vi "Initialize Text Log File.vi"(8 "error in (no error)":errorcluster, 9 "Operation":T1, 10 "File Path":path, 11 "Text Log File Specification in":refnum<class "Text Log File Specification.lvclass">) -> (0 "error out":errorcluster, 1 "Log File out":refnum<class "Log File.lvclass">, 3 "Text Log File Specification out":refnum<class "Text Log File Specification.lvclass">)   [LabVIEW 2015, in "Text Log File Specification.lvclass"]
uses:
  Text Log File Specification.lvclass
  Logs/Log Files/Log File/Log File.lvclass
  Logs/Log Files/Log File/Operation.ctl
  Text Log File Specification.lvclass/Text Log File Specification.ctl
  Logs/Log Files/Text Log File/Text Log File.lvclass
  Logs/Log Files/Text Log File/Text Log File.lvclass/Text Log File.ctl
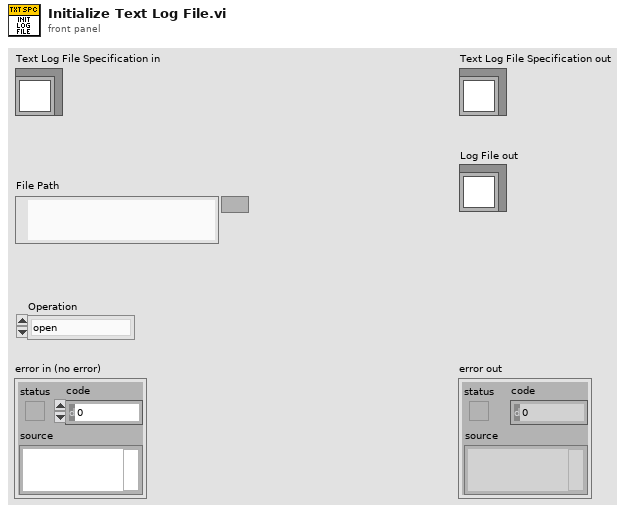
[diagram p1: front panel]
types:
  T1 = typedef "Log File.lvclass/Operation.ctl" = enum16{"open", "open or create", "create or replace", "create", "open (read-only)"}
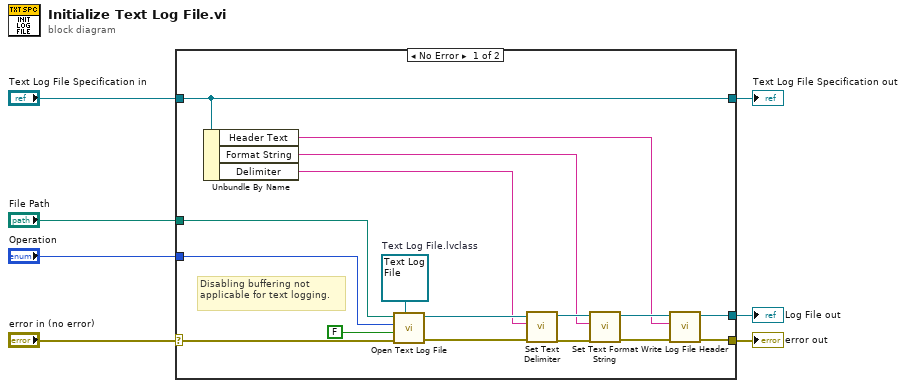
[diagram p0: block diagram]
diagram:
  n1 = case shown="No Error" "error in (no error)" {
    selector: "error in (no error)" -> [w14 w25]
    tunnel: "Text Log File Specification in" -> [w16 w26]
    tunnel: [w16 w26] -> w6
    tunnel: [w9 w25] -> w5
    tunnel: [w10 _] -> w4
    tunnel: "File Path" -> [w15 _]
    tunnel: "Operation" -> [w18 _]
    frame No Error {
      w22 = refnum<class "Text Log File.lvclass"> refnum  # Text Log File.lvclass
      # "Disabling buffering not applicable for text logging."
      n2 = Unbundle By Name(w16) -> ("Header Text"=w8:string, "Format String"=w19:string, "Delimiter"=w17:string)
      n3 = call "Open Text Log File.vi"("Text Log File Type"=w22, "error in (no error)"=w14, "Disable Buffering (F)"=FALSE, "Operation"=w18, "File Path"=w15) -> ("error out"=w20:errorcluster, "Text Log File out"=w21:refnum<class "Text Log File.lvclass">)  [unwired: 5 in]
      n4 = call "Set Text Delimiter.vi"("error in (no error)"=w20, "Delimiter"=w17, "Text Log File in"=w21) -> ("error out"=w23:errorcluster, "Text Log File out"=w24:refnum<class "Text Log File.lvclass">)  [unwired: 7 in]
      n5 = call "Set Text Format String.vi"("error in (no error)"=w23, "Format String"=w19, "Text Log File in"=w24) -> ("error out"=w11:errorcluster, "Text Log File out"=w12:refnum<class "Text Log File.lvclass">)  [unwired: 7 in]
      n6 = call "Write Log File Header.vi"("error in (no error)"=w11, "Header Text"=w8, "Text Log File in"=w12) -> ("error out"=w9:errorcluster, "Text Log File out"=w10:refnum<class "Text Log File.lvclass">)  [unwired: 7 in]
    }
    frame Error {
    }
  }
  "error out" <- w5
  "Text Log File Specification out" <- w6
  "Log File out" <- w4
